vi "Obtain References.vi"(8 "Error In":errorcluster, 9 "grouping":string, 10 "colorMap":string, 11 "VI in":refnum<vi>) -> (0 "Error Out":errorcluster, 3 "Front Panel Objects":refnum<vi>[](array[refnum]))   [LabVIEW 2019, in "LSS.lvlib"]
doc: "This VI obtains a reference to every object on the front panel of the VI reference passed to it. This is used at the start of all applications using LSS to obtain the references it will use later for changing style programatically.\n\n<b>Inputs:</b>\n<b>VI in</b> - Reference to the VI whose front panel will be modified by subsequent LSS calls.\n<b>colorMap</b> - This string is an LSS formatted string that allows the mapping of hexidecimal color constants to string names that are easier to remember. Once a color is defined in the colorMap, any subsequent LSS call can simply use the name of the color instead of the hexidecimal representation. The format for this string is as follows:\n colorMap{\n myColorName:#000000;\n}\n<b>grouping</b> - Style sheet determining how objects will be grouped. The format of the style sheet for grouping objects is as follows:\ngrouping{\n objectGroupName:frontPanelObjectName;\n objectGroupName2:frontPanelObjectName2;\n}\nWhere the specifier grouping must stay the same. objectGroupName is the name of the group, for example \"Group 1\". frontPanelObjectName is the name of the item on the front panel, for example \"Stop Button\". To add two buttons to group alpha would look as follows:\ngrouping{\n group alpha:Start Button;\n group alpha:Stop Button;\n}\n<b>Error In</b> - Error input terminal\n\n<b>Outputs:</b>\n<b>Front Panel Objects</b> - Contains the reference to every front panel object. This reference array must be passed to other LSS function calls.\n<b>Error Out</b> - Error output terminal"
uses:
  LSS.lvlib
  <vilib>/Utility/traverseref.llb/TRef TravTarget.ctl
  Controls/Mode.ctl
  <vilib>/Utility/traverseref.llb/VI Scripting - Traverse.lvlib
panel:
  out "Selectors":string[][](array[string])
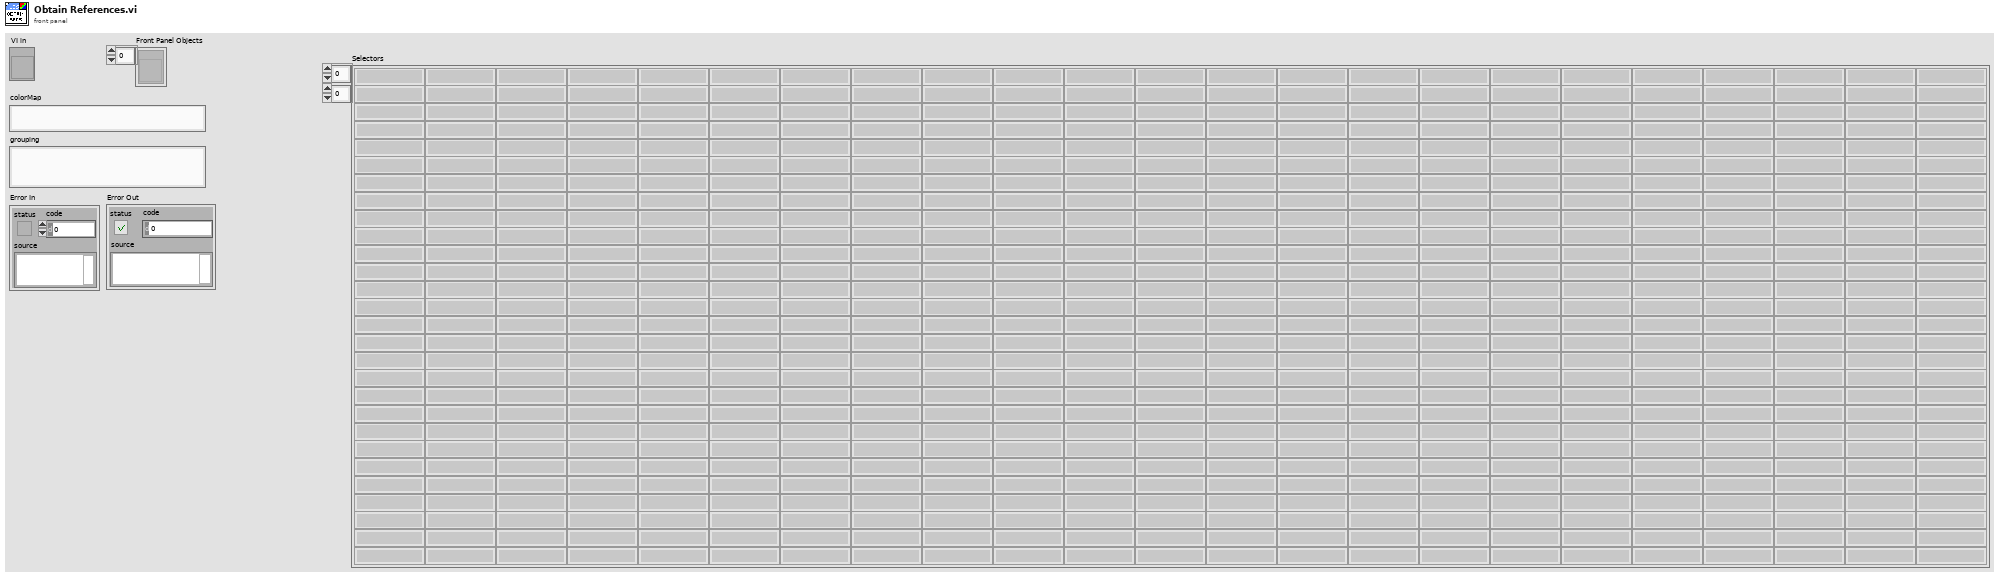
[diagram p1: front panel]
types:
  T1 = typedef "TRef TravTarget.ctl" = enum16{"FP", "BD", "Other"}
  T2 = typedef "LSS.lvlib/Mode.ctl" = enum16{"Write", "Add", "Read"}
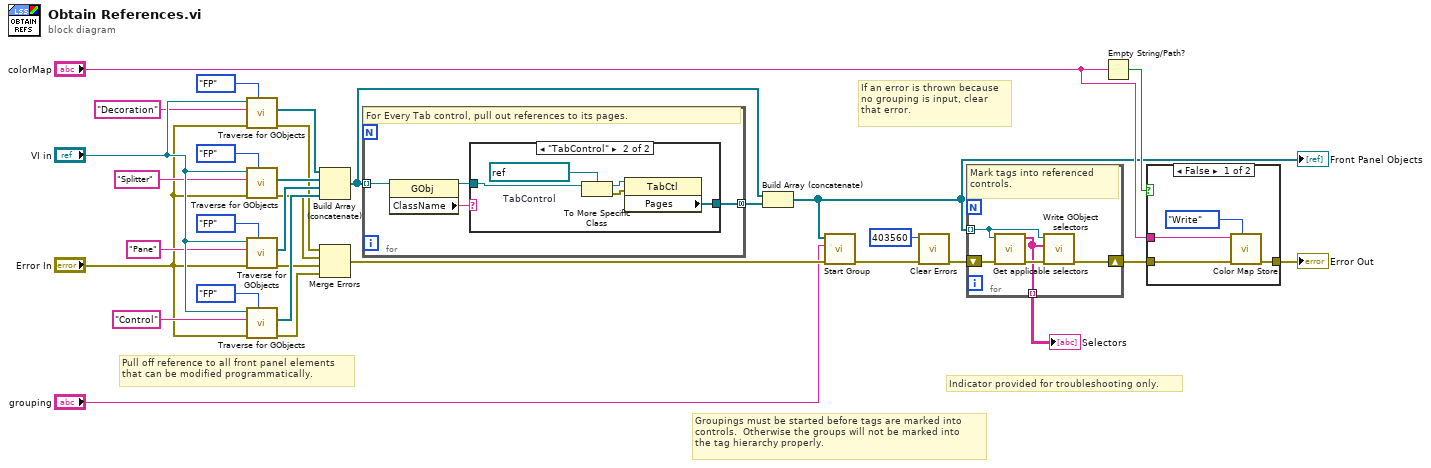
[diagram p0: block diagram]
diagram:
  # "If an error is thrown because\nno grouping is input, clear \nthat error."
  # "Groupings must be started before tags are marked into\ncontrols.  Otherwise the groups will not be marked into\nthe tag hierarchy properly."
  # "Indicator provided for troubleshooting only."
  # "Pull off reference to all front panel elements\nthat can be modified programmatically."
  n1 = call <vilib>:"Traverse for GObjects.vi"("Traverse Target"=TRef_TravTarget."FP", "error in (no error)"="Error In", "Class Name"="Decoration", "VI Refnum"="VI in") -> ("error out"=w18:errorcluster, "References"=w22:refnum<vi>[])  [unwired: 4 in, 2 out]
  n2 = call <vilib>:"Traverse for GObjects.vi"("Traverse Target"=TRef_TravTarget."FP", "error in (no error)"="Error In", "Class Name"="Splitter", "VI Refnum"="VI in") -> ("error out"=w17:errorcluster, "References"=w21:refnum<vi>[])  [unwired: 4 in, 2 out]
  n3 = call <vilib>:"Traverse for GObjects.vi"("Traverse Target"=TRef_TravTarget."FP", "error in (no error)"="Error In", "Class Name"="Pane", "VI Refnum"="VI in") -> ("error out"=w16:errorcluster, "References"=w20:refnum<vi>[])  [unwired: 4 in, 2 out]
  n4 = call <vilib>:"Traverse for GObjects.vi"("Traverse Target"=TRef_TravTarget."FP", "error in (no error)"="Error In", "Class Name"="Control", "VI Refnum"="VI in") -> ("error out"=w15:errorcluster, "References"=w19:refnum<vi>[])  [unwired: 4 in, 2 out]
  n5 = Build Array (concatenate)(w22, w21, w20, w19) -> (w9:refnum<vi>[])
  n6 = Merge Errors(w18, w17, w16, w15) -> (w5:errorcluster)
  n7 = for {
    tunnel: w9 -> [w35] mode=indexing
    tunnel: [w32] -> w8 mode=concatenating
    # "For Every Tab control, pull out references to its pages."
    n8 = property class="GObj"(reference=w35) -> (reference out=w33:refnum<vi>, "ClassName"=w34:string)  [unwired: 1 in, 1 out]
    n9 = case shown="\"TabControl\"" w34 {
      tunnel: w33 -> [_ w40]
      tunnel: [_ w36] -> w32
      frame "False", Default {
      }
      frame "TabControl" {
        w39 = refnum<vi> refnum  # TabControl
        n10 = To More Specific Class(target class=w39, reference=w40) -> (specific class reference=w38:refnum<vi>, error out=w37:errorcluster)  [unwired: 1 in]
        n11 = property class="TabCtl"(reference=w38, error in=w37) -> ("Pages"=w36:refnum<vi>[])  [unwired: 2 out]
      }
    }
  }
  n12 = Build Array (concatenate)(w9, w8) -> (w4:refnum<vi>[])
  "Front Panel Objects" <- w4
  n13 = call "Start Group.vi"("Error In"=w5, "Style Sheet"="grouping", "Front Panel Objects"=w4) -> ("Error Out"=w6:errorcluster)  [unwired: 8 in]
  n14 = call <vilib>:"Clear Errors.vi"("error in (no error)"=w6, "specific error code to clear (0: all)"=403560) -> ("error out"=w2:errorcluster)  [unwired: 4 in, 1 out]
  n15 = for {
    tunnel: w4 -> [w45] mode=indexing
    shift-right: [w43] -> w13
    shift-left: w2 -> [w42]
    tunnel: [w41] -> w7 mode=indexing
    # "Mark tags into referenced controls."
    n16 = call "Get applicable selectors.vi"("Error in"=w42, "GObject"=w45) -> ("Error out"=w44:errorcluster, "Selectors"=w41:string[])  [unwired: 8 in]
    n17 = call "Write GObject selectors.vi"("Error in"=w44, "Selectors"=w41, "GObject in"=w45) -> ("Error out"=w43:errorcluster)  [unwired: 8 in]
  }
  "Selectors" <- w7
  n18 = Empty String/Path?(string/path="colorMap") -> (empty?=w10:bool)
  n19 = case shown="False" w10 {
    tunnel: w13 -> [w48 w50]
    tunnel: [w47 w50] -> w12
    tunnel: "colorMap" -> [w46 _]
    frame False {
      n20 = call "Color Map Store.vi"("Mode"=Mode."Write", "Error In"=w48, "colorMap"=w46) -> ("Error Out"=w47:errorcluster)  [unwired: 6 in, 2 out]
    }
    frame True {
    }
  }
  "Error Out" <- w12
